vi "getCategoryUpdateQuery.vi"(8 "error in (no error)":errorcluster, 10 "Category ID":string, 11 "Credit Transaction in":refnum<class "Credit Transaction.lvclass">) -> (0 "error out":errorcluster, 2 "Update Query":string, 3 "Credit Transaction out":refnum<class "Credit Transaction.lvclass">)   [LabVIEW 2018, in "Credit Transaction.lvclass"]
uses:
  Credit Transaction.lvclass
  Transaction/Transaction.lvclass
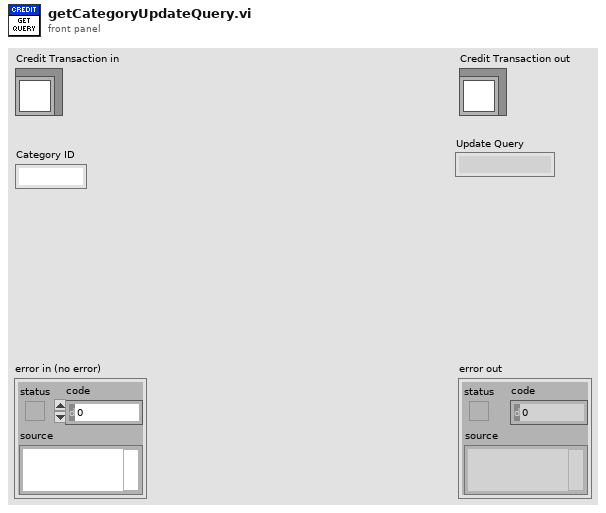
[diagram p1: front panel]
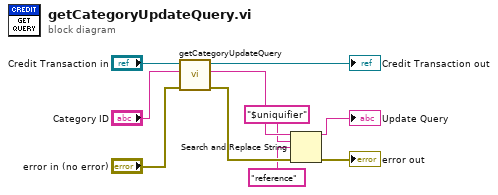
[diagram p0: block diagram]
diagram:
  n1 = call-parent "getCategoryUpdateQuery.vi"("error in (no error)"="error in (no error)", "Category ID"="Category ID", "Transaction in"="Credit Transaction in") -> ("error out"=w10:errorcluster, "Update Query"=w9:string, "Transaction out"=→"Credit Transaction out":refnum<class "Credit Transaction.lvclass">)  [unwired: 6 in]
  n2 = Search and Replace String(input string=w9, search string="$uniquifier", replace string="reference" ("replace string (\"\")"), error in=w10) -> (result string=→"Update Query":string, error out=→"error out":errorcluster)  [unwired: 4 in, 2 out]
